vi "Initialize Front Panel.vi"(8 "error in (no error)":errorcluster, 11 "BoundViewManager in":refnum<class "BoundViewManager.lvclass">) -> (0 "error out":errorcluster, 3 "BoundViewManager out":refnum<class "BoundViewManager.lvclass">)   [LabVIEW 2020, in "BoundViewManager.lvlib" / "BoundViewManager.lvclass"]
doc: "<License>\nCopyright © 2017 Composed Systems, LLC | All rights reserved\nwww.composed.io\n\nAuthor: Ethan Stern <ethan.stern@composed.io>\n\nThis software is provided \"AS IS\" WITHOUT WARRANTIES, either express or implied, AND IS FOR EDUCATIONAL PURPOSES ONLY.\n</License>"
uses:
  <vilib>/gpm_packages/@cs/ViewManager/source/BoundViewManager/BoundViewManager.lvclass
  <vilib>/gpm_packages/@cs/ViewManager/source/BoundViewManager/BoundViewManager.lvclass/BoundViewManager.ctl
  <vilib>/ActorFramework/Message Enqueuer/Message Enqueuer.lvclass
  <vilib>/gpm_packages/@cs/lookup-table/Source/LookupTable/LookupTable.lvclass/LookupTable.ctl
  <vilib>/gpm_packages/@cs/mva-viewable/Source/IViewable/IViewable Messages/Insert Front Panel Msg/Insert Front Panel Msg.lvclass/Insert Front Panel Msg.ctl
  <vilib>/ActorFramework/Message Enqueuer/Message Enqueuer.lvclass/Message Enqueuer.ctl
  61cc6e39-6280-4a2f-9646-d72848929907.vi
  <vilib>/ActorFramework/Message Enqueuer/Enqueue.vi
  <vilib>/gpm_packages/@cs/lookup-table/Source/LookupTable/Read Table Reference.vi
  61cc6e39-6280-4a2f-9646-d72848929907.vi/ab370e2b-ffe5-401e-8971-e7629b4e0087.vi
  <vilib>/gpm_packages/@cs/mva-viewable/Source/IViewable/IViewable Messages/Insert Front Panel Msg/Insert Front Panel Msg.lvclass
  C:/Program Files/National Instruments/LabVIEW 2020/vi.lib/ActorFramework/Message/Message.lvclass
  <vilib>/ActorFramework/Message Priority Queue/Priority Enqueue.vi
  <vilib>/gpm_packages/@cs/mva-viewable/Source/IViewManager/IViewManager/IViewManager.lvclass
  <vilib>/gpm_packages/@cs/lookup-table/Source/LookupTable/LookupTable.lvclass
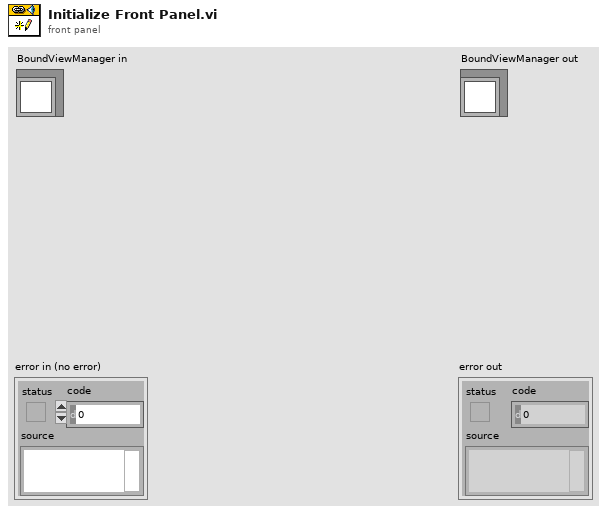
[diagram p1: front panel]
types:
  T1 = typedef "IViewable.lvlib/ProtectedSubpanel.lvclass/Protected Subpanel Reference.ctl" = refnum<data-value>
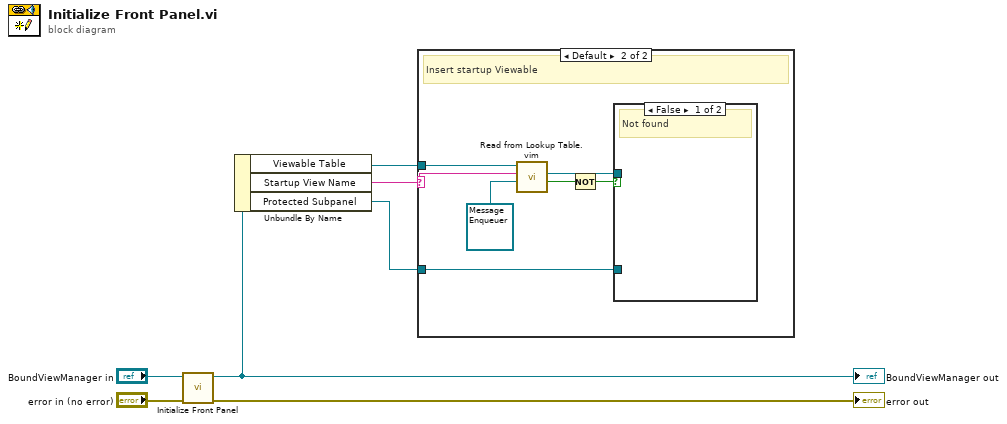
[diagram p0: block diagram]
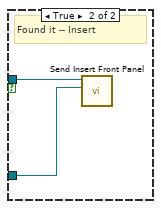
[diagram p3: hidden frame]
diagram:
  n1 = call-parent "Initialize Front Panel.vi"("error in (no error)"="error in (no error)", "IViewable in"="BoundViewManager in") -> ("error out"=→"error out":errorcluster, "IViewable out"=w4:refnum<class "BoundViewManager.lvclass">)  [unwired: 8 in]
  "BoundViewManager out" <- w4
  n2 = Unbundle By Name(w4) -> ("Viewable Table"=w2:refnum<data-value>, "Startup View Name"=w3:string, "Protected Subpanel"=w1:T1)
  n3 = case shown="Default" w3 {
    selector: w3 -> [_ w13]
    tunnel: w2 -> [_ w14]
    tunnel: w1 -> [_ w10]
    frame "" {
      # "No startup viewable insertion"
    }
    frame Default {
      # "Insert startup Viewable"
      n4 = call "Read from Lookup Table.vim"("Type"=refnum<class "Message Enqueuer.lvclass"> refnum ("Message Enqueuer"), "Item Name"=w13, "LookupTable Reference"=w14) -> ("Not Found?"=w12:bool, "Value"=w11:refnum<class "Message Enqueuer.lvclass">)  [unwired: 5 in, 2 out]
      n5 = Not(x=w12) -> (.not. x?=w8:bool)
      n6 = case shown="False" w8 {
        tunnel: w11 -> [_ w15]
        tunnel: w10 -> [_ w16]
        frame False {
          # "Not found"
        }
        frame True {
          # "Found it -- Insert"
          n7 = call <vilib>:"Send Insert Front Panel.vi"("Protected Subpanel"=w16, "Message Enqueuer"=w15) -> ()  [unwired: 8 in, 2 out]
        }
      }
    }
  }
